vi "Publish.vi"(8 "error in (no error)":errorcluster, 9 "Payload":variant, 10 "Topic Name (empty: Payload name)":string, 11 "MQTT_Base in":refnum<class "MQTT_Base.lvclass">) -> (0 "error out":errorcluster, 3 "MQTT_Base out":refnum<class "MQTT_Base.lvclass">)   [LabVIEW 2013, in "MQTT Server.lvlib" / "MQTT_Base.lvclass"]
uses:
  MQTT_Base.lvclass
  <vilib>/LabVIEW Open Source Project/Configuration Manager/Serializer/Serializer.lvclass
  <vilib>/LabVIEW Open Source/Data Manipulation/TypeDescriptor/TypeDescriptor_GetName.vi
  <vilib>/LabVIEW Open Source/Data Manipulation/TypeDescriptor/TypeDescriptor_GetPString.vi
  Control Packets/PUBLISH/PUBLISH.lvclass
  <vilib>/LabVIEW Open Source/Data Manipulation/Variant/OpenVariant.lvlib
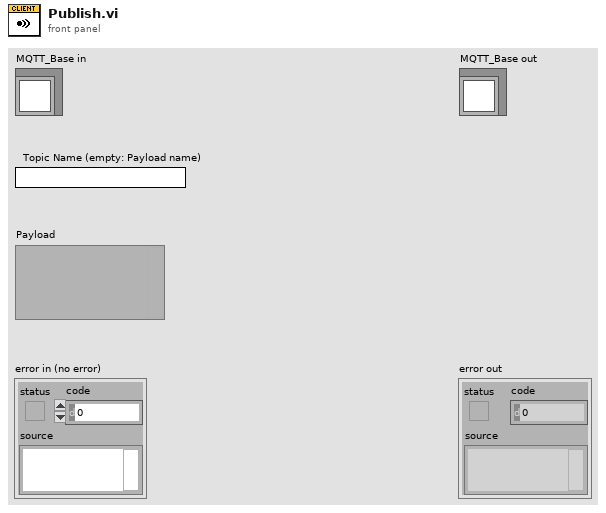
[diagram p1: front panel]
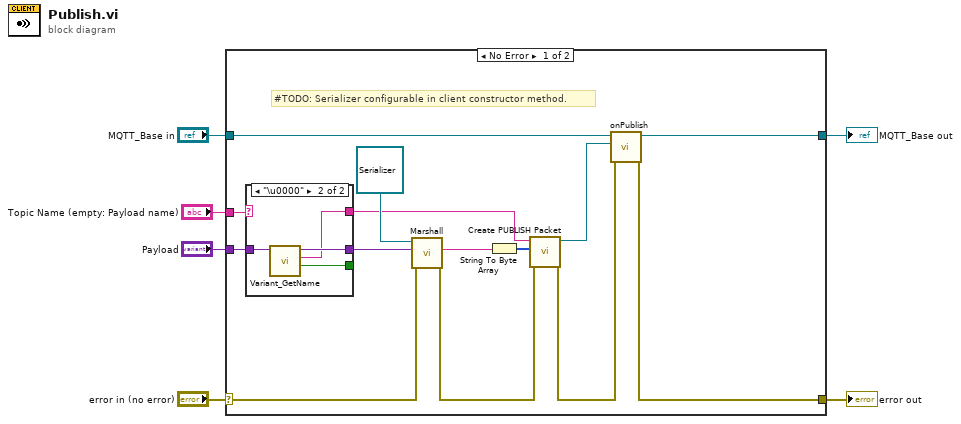
[diagram p0: block diagram]
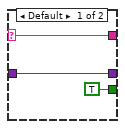
[diagram p2: hidden frame]
diagram:
  n1 = case shown="No Error" "error in (no error)" {
    selector: "error in (no error)" -> [w10 w29]
    tunnel: [w9 w29] -> w5
    tunnel: [w8 w28] -> w3
    tunnel: "MQTT_Base in" -> [w7 w28]
    tunnel: "Payload" -> [w16 _]
    tunnel: "Topic Name (empty: Payload name)" -> [w14 _]
    frame No Error {
      # "#TODO: Serializer configurable in client constructor method."
      n2 = case shown="\"\"" w14 {
        selector: w14 -> [w23 _]
        tunnel: w16 -> [w22 w27]
        tunnel: [w22 w26] -> w15
        tunnel: [w23 w25] -> w13
        tunnel: [TRUE ("found") w24] -> _
        frame Default {
        }
        frame "\u0000" {
          n3 = call <vilib>:"Variant_GetName.vi"("Variant"=w27) -> ("found"=w24:bool, "Name"=w25:string, "Variant dup"=w26:variant)  [unwired: 8 in]
        }
      }
      n4 = call-dynamic "Marshall.vi"("error in (no error)"=w10, "Variant"=w15, "Serializer in"=refnum<class "Serializer.lvclass"> refnum) -> ("error out"=w12:errorcluster, "String"=w19:string)  [unwired: 6 in, 1 out]
      n5 = String To Byte Array(string=w19) -> (unsigned byte array=w18:u8[])
      n6 = call "Create PUBLISH Packet.vi"("error in (no error)"=w12, "Payload"=w18, "Topic Name"=w13) -> ("error out"=w11:errorcluster, "PUBLISH"=w20:refnum<class "PUBLISH.lvclass">)  [unwired: 6 in, 1 out]
      n7 = call-dynamic "onPublish.vi"("error in (no error)"=w11, "PUBLISH"=w20, "MQTT_Base in"=w7) -> ("error out"=w9:errorcluster, "MQTT_Base out"=w8:refnum<class "MQTT_Base.lvclass">)  [unwired: 7 in]
    }
    frame Error {
    }
  }
  "error out" <- w5
  "MQTT_Base out" <- w3
